vi "PropertyChangedEventCallbackForBufferIndexDroppedFramesDiskStreamQueueSize.vi"(4 "User Parameter":cluster{refnum<vi>, refnum<vi>, refnum<vi>}, 5 "Event Data":cluster{"sender":refnum<k24>, "e":refnum<k24>}, 6 "Control Ref":refnum<k24>, 7 "Event Common Data":T1) -> ()   [LabVIEW 2020]
uses:
  C:/Users/Public/Documents/Photometrics/PMQI-LabViewSamples/Examples/2018/Dependencies/PVCamNET.dll
  Dependencies/PVCamNET.dll
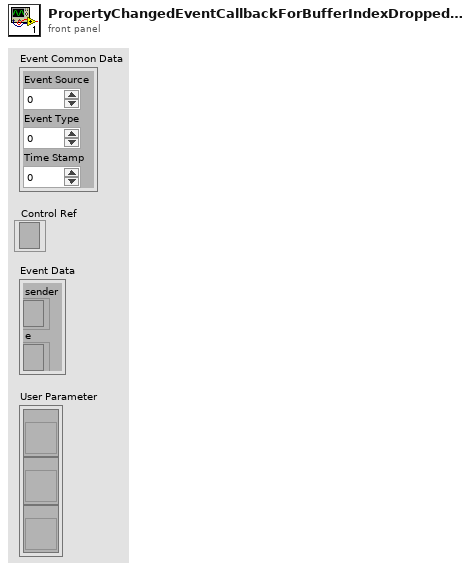
[diagram p1: front panel]
types:
  T1 = cluster{"Event Source":i32, "Event Type":u32, "Time Stamp":u32}
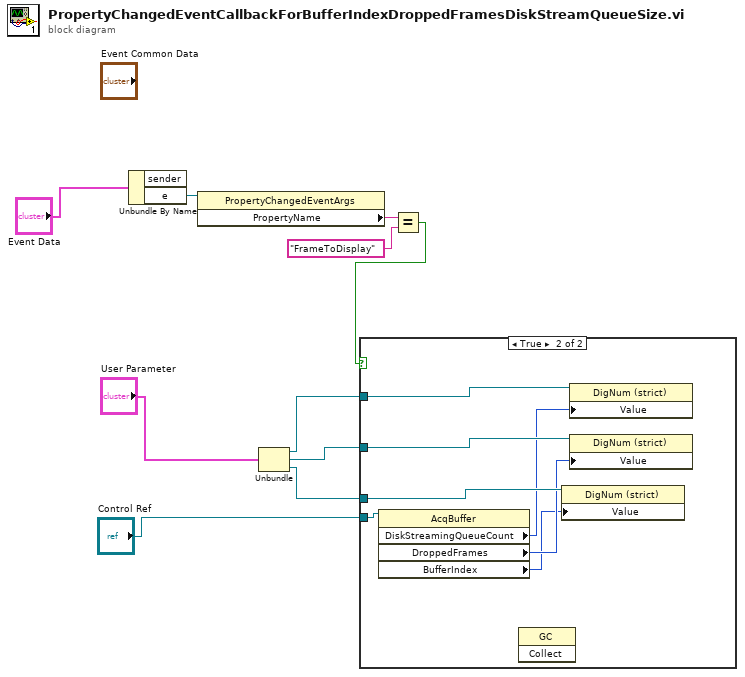
[diagram p0: block diagram]
diagram:
  n1 = Unbundle By Name("Event Data") -> ("e"=w5:refnum<k24>)  [unwired: 1 out]
  n2 = property class="PropertyChangedEventArgs"(reference=w5) -> ("PropertyName"=w4:string)  [unwired: 1 in, 2 out]
  n3 = Unbundle("User Parameter") -> (w10:refnum<vi>, w9:refnum<vi>, w8:refnum<vi>)
  n4 = Equal?(x=w4, y="FrameToDisplay") -> (x = y?=w1:bool)
  n5 = case shown="True" w1 {
    tunnel: w10 -> [_ w17]
    tunnel: "Control Ref" -> [_ w16]
    tunnel: w9 -> [_ w15]
    tunnel: w8 -> [_ w14]
    frame False {
    }
    frame True {
      n6 = property class="AcqBuffer"(reference=w16) -> ("DiskStreamingQueueCount"=w13:u32, "DroppedFrames"=w12:u32, "BufferIndex"=w11:u32)  [unwired: 1 in, 2 out]
      n7 = invoke class="GC" method="Collect"() -> ()  [unwired: 3 in, 3 out]
      n8 = property class="DigNum (strict)"(reference=w14, "Value"=w11) -> ()  [unwired: 1 in, 2 out]
      n9 = property class="DigNum (strict)"(reference=w17, "Value"=w13) -> ()  [unwired: 1 in, 2 out]
      n10 = property class="DigNum (strict)"(reference=w15, "Value"=w12) -> ()  [unwired: 1 in, 2 out]
    }
  }
